vi "ts2Polo.vi"(8 "Tm":dbl, 10 "Tao":dbl, 11 "Epsilon":dbl) -> (2 "Plano Z":cluster{"X":dbl, "Y":dbl}[](graph), 4 "Polos (Z1,Z2)":cdb[](array[numeric]) format="%#_3g", 5 "F(z)":dbl[](array[numeric]))   [LabVIEW 2020]
doc: "Calcula y grafica los polos de un sistema discreto de segundo orden, a partir de la constante de tiempo (Tao), del coeficiente de amortiguamiento (Epsilon) y del periodo de muestreo (Tm).\n\nPor \nJuan David Núñez López\nIng. Instrumentación y Control"
uses:
  <vilib>/Analysis/polynomials.llb/Create Polynomial From Roots (CDB).vi
  <vilib>/Analysis/NI_AALPro.lvlib
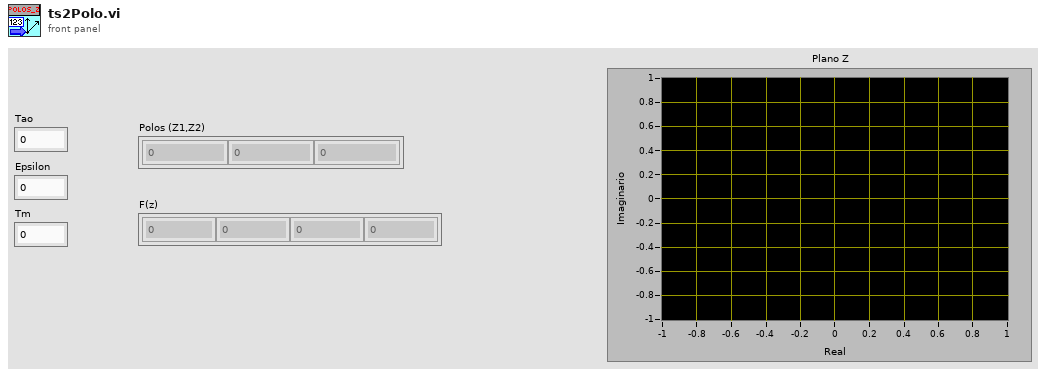
[diagram p1: front panel]
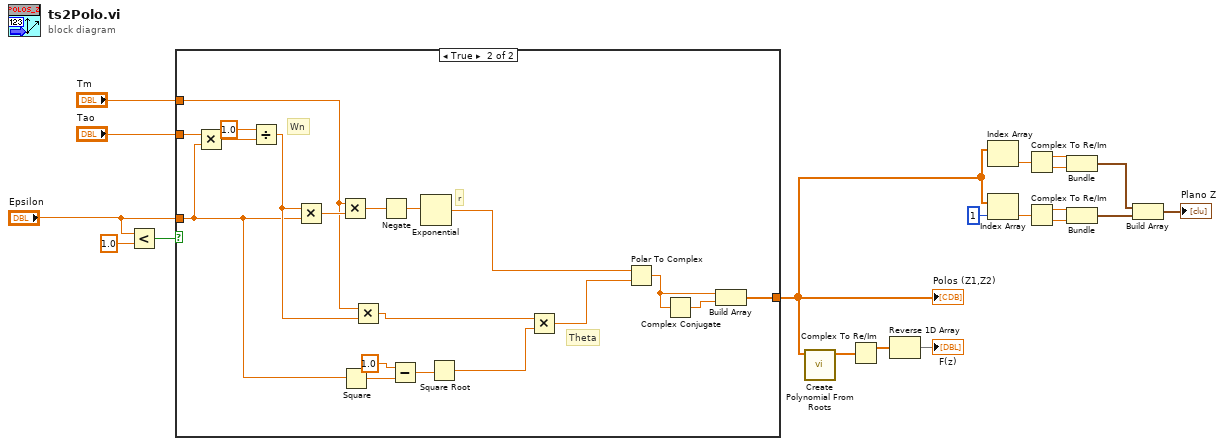
[diagram p0: block diagram]
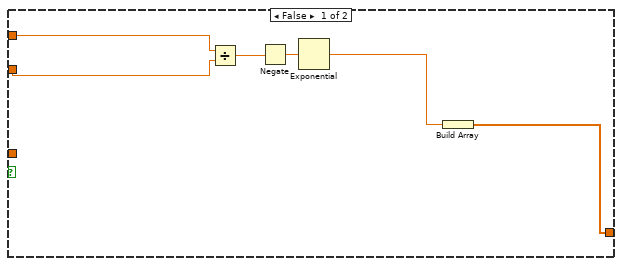
[diagram p2: hidden frame]
diagram:
  n1 = Less?(x="Epsilon", y=1.0) -> (x < y?=w18:bool)
  n2 = case shown="True" w18 {
    tunnel: "Tao" -> [w22 w44]
    tunnel: [w20 w32] -> w1
    tunnel: "Tm" -> [w23 w31]
    tunnel: "Epsilon" -> [_ w30]
    frame False {
      n3 = Divide(x=w23, y=w22) -> (x/y=w24:dbl)
      n4 = Negate(x=w24) -> (-x=w25:dbl)
      n5 = Exponential(1:w25) -> (0:w21:dbl)
      n6 = Build Array(w21) -> (w20:dbl[])
    }
    frame True {
      # "Theta"
      # "Wn"
      # "r"
      n7 = Multiply(x=w44, y=w30) -> (x*y=w28:dbl)
      n8 = Divide(x=1.0, y=w28) -> (x/y=w40:dbl)
      n9 = Multiply(x=w40, y=w30) -> (x*y=w43:dbl)
      n10 = Multiply(x=w31, y=w43) -> (x*y=w42:dbl)
      n11 = Square(x=w30) -> (x^2=w39:dbl)
      n12 = Multiply(x=w31, y=w40) -> (x*y=w26:dbl)
      n13 = Negate(x=w42) -> (-x=w41:dbl)
      n14 = Subtract(x=1.0, y=w39) -> (x-y=w37:dbl)
      n15 = Exponential(1:w41) -> (0:w35:dbl)
      n16 = Square Root(x=w37) -> (sqrt(x)=w36:dbl)
      n17 = Multiply(x=w26, y=w36) -> (x*y=w29:dbl)
      n18 = Polar To Complex(1:w29, 2:w35) -> (0:w34:cdb)
      n19 = Complex Conjugate(1:w34) -> (0:w33:cdb)
      n20 = Build Array(w34, w33) -> (w32:cdb[])
    }
  }
  "Polos (Z1,Z2)" <- w1
  n21 = call-poly <vilib>:"Create Polynomial From Roots.vi"("Roots"=w1) -> ("P(x)"=w14:cdb[])  [unwired: 9 in, 1 out]
  n22 = Complex To Re/Im(x + iy=w14) -> (x=w13:dbl[])  [unwired: 1 out]
  n23 = Reverse 1D Array(array=w13) -> (reversed array=→"F(z)":dbl[])
  n24 = Index Array(array=w1) -> (element=w10:cdb)  [unwired: 1 in]
  n25 = Index Array(array=w1, index=1) -> (element=w11:cdb)
  n26 = Complex To Re/Im(x + iy=w10) -> (x=w5:dbl, y=w4:dbl)
  n27 = Complex To Re/Im(x + iy=w11) -> (x=w3:dbl, y=w2:dbl)
  n28 = Bundle(w5, w4) -> (w8:cluster{dbl, dbl})  [unwired: 1 in]
  n29 = Bundle(w3, w2) -> (w6:cluster{dbl, dbl})  [unwired: 1 in]
  n30 = Build Array(w8, w6) -> (→"Plano Z":cluster{dbl, dbl}[])
